vi "Get Dependencies.vi"(11 "GPack File in":refnum<class "GPack File.lvclass">) -> (2 "Dependencies":T1[](array[typedef]))   [LabVIEW 2020, in "GPack.lvlib" / "GPack File.lvclass"]
uses:
  GPack File.lvclass
  Dependency.ctl
  Package Info.ctl
  GPack File.lvclass/GPack File.ctl
  GPack.lvlib
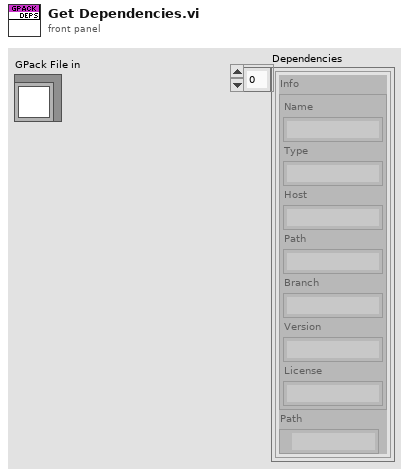
[diagram p1: front panel]
types:
  T1 = typedef "GPack.lvlib/Dependency.ctl" = cluster{"Info":T2, "Path":path}
  T2 = typedef "GPack.lvlib/Package Info.ctl" = cluster{"Name":string, "Type":string, "Host":string, "Path":string, "Branch":string, "Version":string, "License":string}
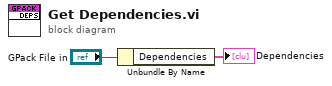
[diagram p0: block diagram]
diagram:
  n1 = Unbundle By Name("GPack File in") -> ("Dependencies"=→"Dependencies":T1[])
